vi "总磷总氮启动参数对话框.vi"() -> (2 "确认":bool, 3 "元素":cluster{"命令":string, "data":variant})   [LabVIEW 2016, in "斯坦道总氮V2.lvlib"]
panel:
  out "标液值":dbl caption="标液值："
  in  "取消":bool
  in  "确定":bool
  in  "量程切换":u16(ring)=2 items=["高量程", "低量程", "自动"]
  in  "站号":u16(ring)=1 items=["氨氮"=3]
  in  "控制命令":T1(ring)
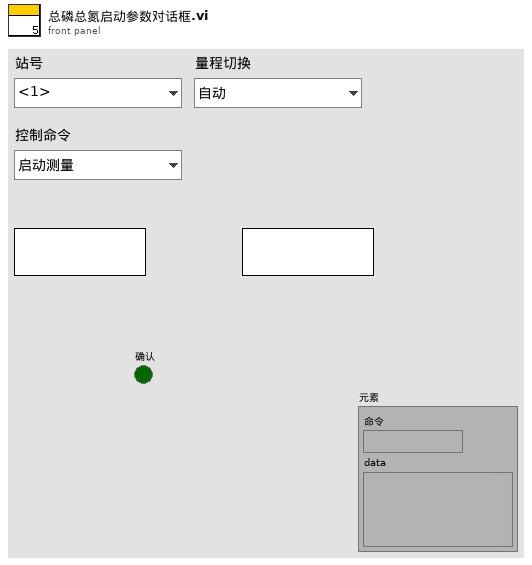
[diagram p1: front panel]
types:
  T1 = enum16{"启动测量", "标样核查", "零点核查", "跨度核查", "空白测试", "平行样测试", "加标回收", "空白校准", "标样校准", "初始化（清洗）", "停止测试", "仪器重启", "校时", "模式设置", "测量间隔设置"}
  T2 = typedef "LVStringsAndValuesArrayTypeDef_U16.ctl" = cluster{"String":string, "Value":u16}[]
  T3 = cluster{"时间标识":timestamp, "设备":string, "日志信息":string, "流程参数":string}
  T4 = cluster{"站号":u16, "量程切换":enum32{"H", "L", "AUTO"}, "控制命令":enum16{"启动测量", "标样核查", "零点核查", "跨度核查", "空白测试", "平行样测试", "加标回收", "空白校准", "标样校准", "初始化（清洗）", "停止测试", "仪器重启", "校时", "模式设置", "测量间隔设置", "盲样测试"}, "模式设置":enum16{"待机", "连续模式", "周期模式", "定点模式", "受控模式", "手动模式"}, "测量间隔":u16}
  T5 = cluster{"总磷跨度值":dbl, "总磷零点标准液浓度":dbl, "总磷跨度标准液浓度":dbl, "总磷标准液标准浓度":dbl, "总氮跨度值":dbl, "总氮零点标准液浓度":dbl, "总氮跨度标准液浓度":dbl, "总氮标准液标准浓度":dbl, "氨氮跨度值":dbl, "氨氮零点标准液浓度":dbl, "氨氮跨度标准液浓度":dbl, "氨氮标准液标准浓度":dbl}
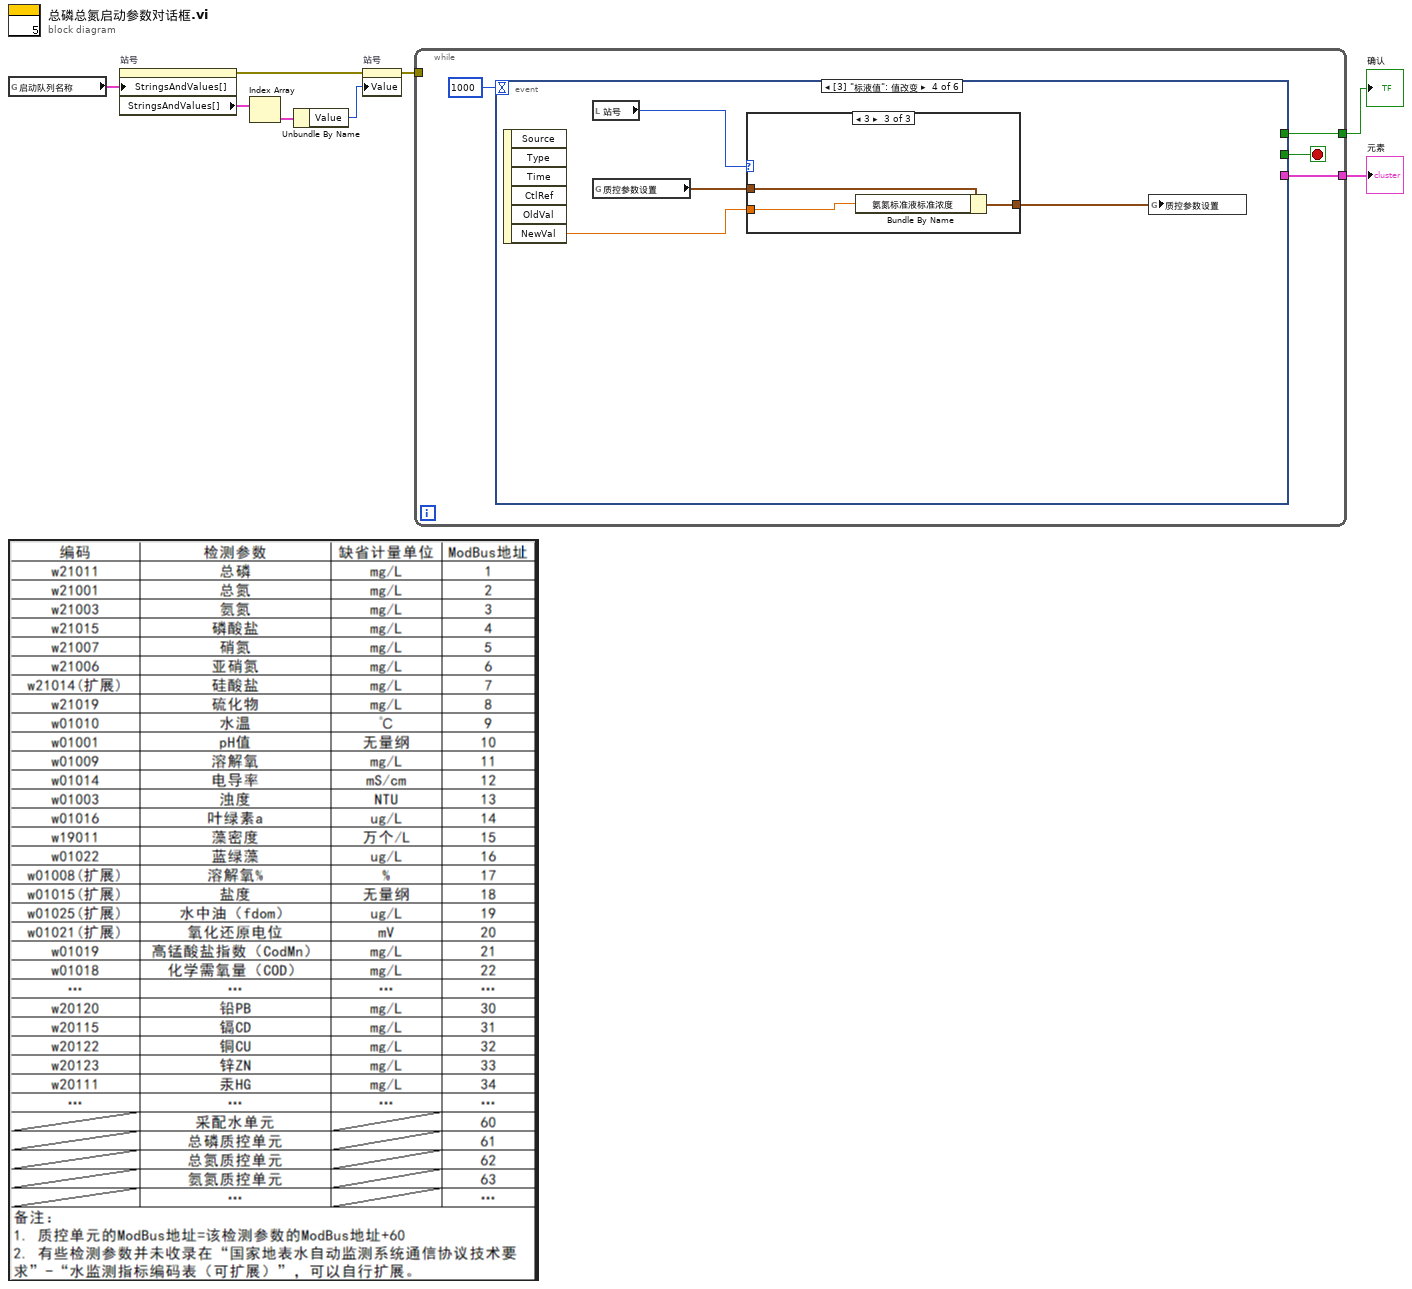
[diagram p0: block diagram]
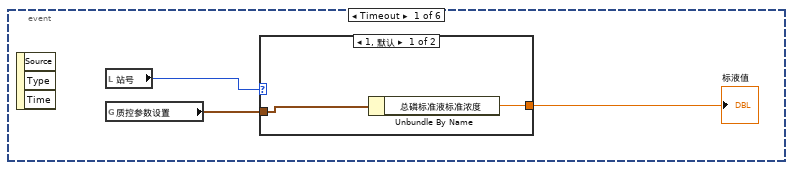
[diagram p2: hidden frame]
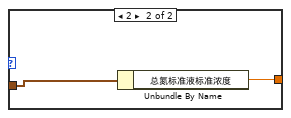
[diagram p3: hidden frame]
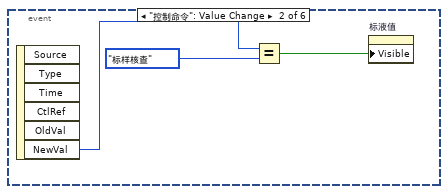
[diagram p4: hidden frame]
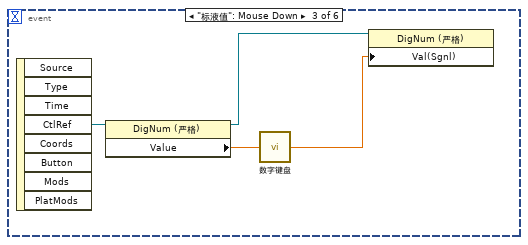
[diagram p5: hidden frame]
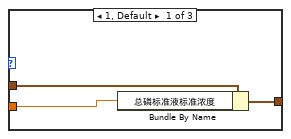
[diagram p6: hidden frame]
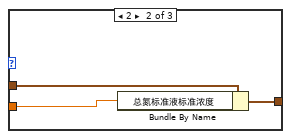
[diagram p7: hidden frame]
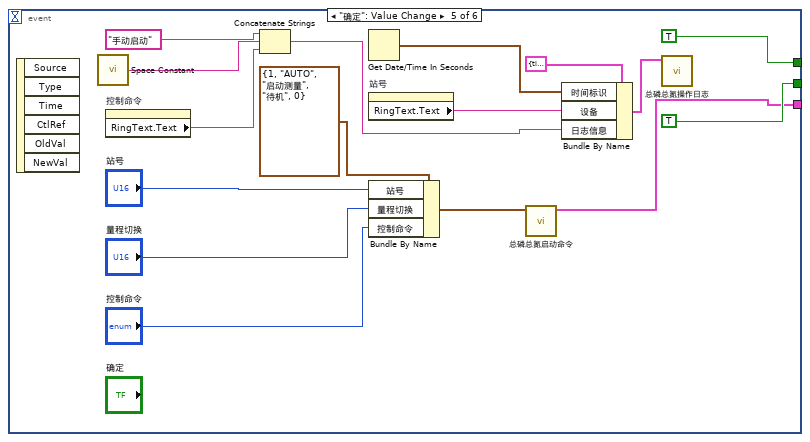
[diagram p8: hidden frame]
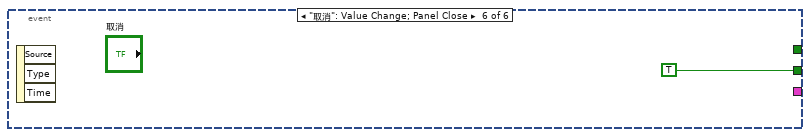
[diagram p9: hidden frame]
diagram:
  n1 = global read "总磷总氮断电保存全局变量.vi" "启动队列名称"() -> (w6:cluster{"String":string, "Value":u16}[])
  n2 = property on="站号" class="Ring (严格)"("StringsAndValues[]"=w6) -> (error out=w5:errorcluster, "StringsAndValues[]"=w4:T2)  [unwired: 2 in, 1 out]
  n3 = Index Array(array=w4) -> (element=w3:cluster{"String":string, "Value":u16})  [unwired: 1 in]
  n4 = Unbundle By Name(w3) -> ("Value"=w2:u16)
  n5 = property on="站号" class="Ring (严格)"(error in=w5, "Value"=w2) -> (error out=w1:errorcluster)  [unwired: 1 in, 1 out]
  n6 = while {
    tunnel: [w10] -> w8
    tunnel: [w9] -> w7
    tunnel: w1 -> [_]
    stop <- w12 stop-if-true
    n7 = event shown="[3] \"标液值\": 值改变" {
      selector: _ -> [_ _ _ _ _ _]
      dyn-events: _ -> [_ _ _ _ _ _]
      timeout: 1000 -> [_ _ _ _ _ _]
      tunnel: [_ _ _ _ TRUE TRUE] -> w12
      tunnel: [_ _ _ _ TRUE _] -> w10
      tunnel: [_ _ _ _ w53 _] -> w9
      event Timeout {
        n8 = event-data() -> ()  [unwired: 1 in, 3 out]
        n9 = local read "站号"() -> (w14:u16)
        n10 = global read "总磷总氮断电保存全局变量.vi" "质控参数设置"() -> (w15:T5)
        n11 = case shown="1, 默认" w14 {
          tunnel: w15 -> [w17 w19]
          tunnel: [w16 w18] -> w13
          frame 1, Default {
            n12 = Unbundle By Name(w17) -> ("总磷标准液标准浓度"=w16:dbl)
          }
          frame 2 {
            n13 = Unbundle By Name(w19) -> ("总氮标准液标准浓度"=w18:dbl)
          }
        }
        "标液值" <- w13
      }
      event "控制命令": Value Change {
        n14 = event-data() -> ("NewVal"=w22:T1)  [unwired: 1 in, 5 out]
        n15 = Equal?(x=w22, y=T1."标样核查") -> (x = y?=w20:bool)
        n16 = property on="标液值" class="DigNum (严格)"("Visible"=w20) -> ()  [unwired: 2 in, 2 out]
      }
      event "标液值": Mouse Down {
        n17 = event-data() -> ("CtlRef"=w26:refnum<vi>)  [unwired: 1 in, 7 out]
        n18 = property class="DigNum (严格)"(reference=w26) -> (reference out=w23:refnum<vi>, "Value"=w25:dbl)  [unwired: 1 in, 1 out]
        n19 = call "数字键盘.vi"("OldNumber"=w25) -> ("NewNumber"=w24:dbl)
        n20 = property class="DigNum (严格)"(reference=w23, "Val(Sgnl)"=w24) -> ()  [unwired: 1 in, 2 out]
      }
      event "标液值": Value Change {
        n21 = event-data() -> ("NewVal"=w28:dbl)  [unwired: 1 in, 5 out]
        n22 = local read "站号"() -> (w30:u16)
        n23 = global read "总磷总氮断电保存全局变量.vi" "质控参数设置"() -> (w29:T5)
        n24 = case shown="3" w30 {
          tunnel: w29 -> [w33 w36 w39]
          tunnel: [w31 w34 w37] -> w27
          tunnel: w28 -> [w32 w35 w38]
          frame 1, Default {
            n25 = Bundle By Name(cluster=w33, "总磷标准液标准浓度"=w32) -> (w31:T5)
          }
          frame 2 {
            n26 = Bundle By Name(cluster=w36, "总氮标准液标准浓度"=w35) -> (w34:T5)
          }
          frame 3 {
            n27 = Bundle By Name(cluster=w39, "氨氮标准液标准浓度"=w38) -> (w37:T5)
          }
        }
        n28 = global write "总磷总氮断电保存全局变量.vi" "质控参数设置"(w27) -> ()
      }
      event "确定": Value Change {
        n29 = event-data() -> ()  [unwired: 1 in, 6 out]
        n30 = call <vilib>:"Space Constant.vi"() -> ("String"=w40:string)
        n31 = property on="控制命令" class="Enum (严格)"() -> ("RingText.Text"=w41:string)  [unwired: 2 in, 2 out]
        n32 = Concatenate Strings("手动启动" ("日志信息"), w40, w41) -> (w42:string)
        n33 = Get Date/Time In Seconds() -> (seconds since 1Jan1904=w46:timestamp)
        n34 = property on="站号" class="Ring (严格)"() -> ("RingText.Text"=w44:string)  [unwired: 2 in, 2 out]
        n35 = Bundle By Name(cluster=T4 {"站号"=1, "量程切换"=enum."AUTO", "控制命令"=enum."启动测量", "模式设置"=enum."待机", "测量间隔"=0} ("参数"), "站号"="站号", "量程切换"="量程切换", "控制命令"="控制命令") -> (w51:T4)
        n36 = call "总磷总氮启动命令.vi"("参数"=w51) -> ("启动命令"=w53:cluster{"命令":string, "data":variant})  [unwired: 10 in]
        n37 = Bundle By Name(cluster=T3 {"时间标识"=timestamp(0 s since 1904-01-01), "设备"="", "日志信息"="", "流程参数"=""} ("data in"), "时间标识"=w46, "设备"=w44, "日志信息"=w42) -> (w45:T3)
        n38 = call "总磷总氮操作日志.vi"("data in"=w45) -> ()  [unwired: 10 in, 1 out]
      }
      event "取消": Value Change; Panel Close {
        n39 = event-data() -> ()  [unwired: 1 in, 3 out]
      }
    }
  }
  "元素" <- w7
  "确认" <- w8
